vi "startNextCycle.vi"(8 "error in (no error)":errorcluster, 11 "Model in":refnum<class "Model.lvclass">) -> (0 "error out":errorcluster, 3 "Model out":refnum<class "Model.lvclass">)   [LabVIEW 2013, in "Model.lvclass"]
uses:
  Model.lvclass
  Model.lvclass/Model.ctl
  ApplicationElements/Log/TestDataLog/TestDataLog.lvclass/TestDataLog.ctl
  UserEvents/UserEvents.lvclass/UserEvents.ctl
  ApplicationElements/TestMonitor/TestMonitor.lvclass
  UserEvents/UserEvents.lvclass
  ApplicationElements/Log/TestDataLog/TestDataLog.lvclass
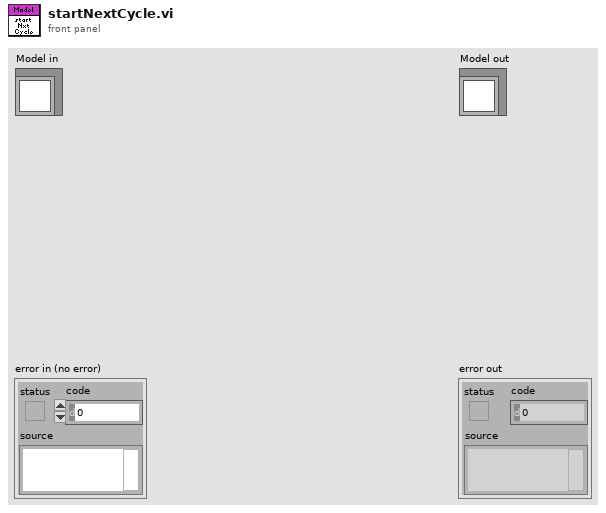
[diagram p1: front panel]
types:
  T1 = typedef "AITDTTypedefs.lvlib/TestStatus.ctl" = cluster{"activeCycle":u32, "activeProfileStep":u32, "demandedCycles":u32, "demandedProfileSteps":u32, "temperatureSetpoint":dbl[unit], "pgaGainCoefficient":u16}
  T2 = typedef "AITDTTypedefs.lvlib/PubDataEvents.ctl" = cluster{"State":refnum<user-event>, "ErrorCode":refnum<user-event>, "OutputData":refnum<user-event>, "InputData":refnum<user-event>, "TestStatus":refnum<user-event>, "LogPath":refnum<user-event>, "TemperatureSetpointRequest":refnum<user-event>, "TemperatureSettling":refnum<user-event>, "WaitTimeStatus":refnum<user-event>}
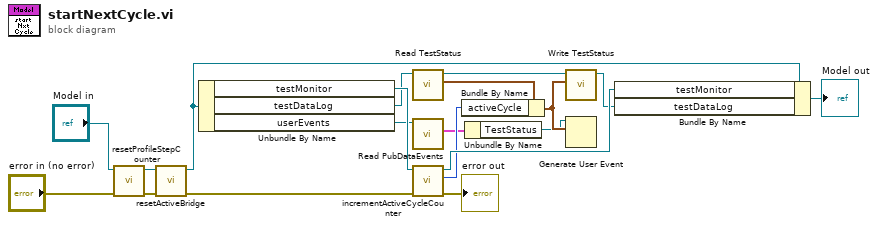
[diagram p0: block diagram]
diagram:
  n1 = call "resetProfileStepCounter.vi"("error in (no error)"="error in (no error)", "Model in"="Model in") -> ("error out"=w3:errorcluster, "Model out"=w4:refnum<class "Model.lvclass">)  [unwired: 8 in]
  n2 = call "resetActiveBridge.vi"("error in (no error)"=w3, "Model in"=w4) -> ("error out"=w1:errorcluster, "Model out"=w2:refnum<class "Model.lvclass">)  [unwired: 8 in]
  n3 = Unbundle By Name(w2) -> ("testMonitor"=w19:refnum<class "TestMonitor.lvclass">, "testDataLog"=w10:refnum<class "TestDataLog.lvclass">, "userEvents"=w5:refnum<class "UserEvents.lvclass">)
  n4 = call "Read TestStatus.vi"("Logger in"=w10) -> ("TestStatus"=w13:T1, "Logger out"=w12:refnum<class "TestDataLog.lvclass">)  [unwired: 9 in]
  n5 = call "Read PubDataEvents.vi"("UserEvents in"=w5) -> ("PubDataEvents"=w7:T2)  [unwired: 9 in, 1 out]
  n6 = call "incrementActiveCycleCounter.vi"("error in (no error)"=w1, "TestMonitor in"=w19) -> ("error out"=→"error out":errorcluster, "activeCycle"=w11:u32, "TestMonitor out"=w14:refnum<class "TestMonitor.lvclass">)  [unwired: 7 in]
  n7 = Bundle By Name(cluster=w13, "activeCycle"=w11) -> (w8:T1)
  n8 = Unbundle By Name(w7) -> ("TestStatus"=w6:refnum<user-event>)
  n9 = call "Write TestStatus.vi"("TestStatus"=w8, "Logger in"=w12) -> ("Logger out"=w9:refnum<class "TestDataLog.lvclass">)  [unwired: 9 in]
  n10 = Generate User Event(user event=w6, event data cluster=w8) -> ()  [unwired: 2 in, 2 out]
  n11 = Bundle By Name(cluster=w2, "testMonitor"=w14, "testDataLog"=w9) -> (→"Model out":refnum<class "Model.lvclass">)
